vi "Set Struct Transfer Mode.vi"(8 "error in":errorcluster, 10 "Allow struct tranfer (False)":bool, 11 "GOLPI ref. in":T1={"pipe handle"={"lv_proc.dll file path"=path "", "process instance handle"=[], "debug mode"=FALSE, "debug data"=[]}, "fast read timeout [ms]"=500, "fast read settle time [ms]"=10, "fast read to multiple [ms]"=1, "max elements per input line"=100, "slow read timeout [ms]"=5000, "stdin double format specifier"="", "max elements per stdout output column"=100, "console mode bitstream"=FALSE, "bitstream first read timeout [ms]"=1000, "bitstream read timeout [ms]"=50, "struct transfer possible"=FALSE}) -> (0 "error out":errorcluster, 2 "conv struct possible?":bool, 3 "GOLPI ref. out":T1={"pipe handle"={"lv_proc.dll file path"=path "", "process instance handle"=[], "debug mode"=FALSE, "debug data"=[]}, "fast read timeout [ms]"=500, "fast read settle time [ms]"=10, "fast read to multiple [ms]"=1, "max elements per input line"=100, "slow read timeout [ms]"=5000, "stdin double format specifier"="", "max elements per stdout output column"=100, "console mode bitstream"=FALSE, "bitstream first read timeout [ms]"=1000, "bitstream read timeout [ms]"=50, "struct transfer possible"=FALSE})   [LabVIEW 2013, in "GOLPI library.lvlib"]
doc: "Set structure transfer mode. This is required for transfering of GNU Octave structures into LabVIEW cluster. First this VI tries to install GNU Octave package golpi. Than package is loaded and VI checks if function golpi_conv_struct() is available in current GNU Octave instance. If not the VIs related to structure tranfer will generate errors. This VI must be called before the structure transfer VIs can be used.\n\n---\nGOLPI works only with lv_proc.dll library, which is part of vipm package or should be delivered together with packed library. Placement of this dll is selected in terminal of Start GNU Octave.vi."
uses:
  GOLPI library.lvlib
  GOLPI reference Type Def.ctl
  LV Process source distribution/Pipe Handle.ctl
  Private/Type Definitions/Custom Error Codes Enum Type Def.vi
  <vilib>/regexp/Match Regular Expression.xnode
  LV Process source distribution/LV Process library.lvlib
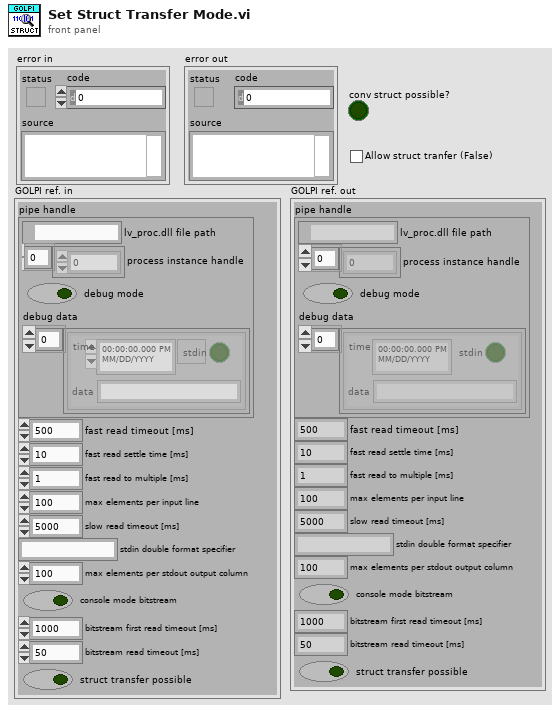
[diagram p1: front panel]
types:
  T1 = typedef "GOLPI library.lvlib/GOLPI reference Type Def.ctl" = cluster{"pipe handle":T2, "fast read timeout [ms]":u32, "fast read settle time [ms]":u32, "fast read to multiple [ms]":u32, "max elements per input line":u32, "slow read timeout [ms]":u32, "stdin double format specifier":string, "max elements per stdout output column":u32, "console mode bitstream":bool, "bitstream first read timeout [ms]":u32, "bitstream read timeout [ms]":u32, "struct transfer possible":bool}
  T2 = typedef "LV Process library.lvlib/Pipe Handle.ctl" = cluster{"lv_proc.dll file path":path, "process instance handle":u32[], "debug mode":bool, "debug data":cluster{"time":timestamp, "stdin":bool, "data":string}[]}
  T3 = typedef "GOLPI library.lvlib/Custom Error Codes Enum Type Def.vi" = enum16{"no error", "00 working directory PAR1 missing", "01 octave binary PAR1 missing", "02 octave report error PAR1", "03 empty output last cmd PAR1", "04 missing temporary file PAR1", "05 pwd PAR 1 not exist", "06 oct package not installed", "10 var PAR1 not string, vect", "11 var PAR1 not num, scal, ~compl", "12 var PAR1 not num, scal, compl", "13 var PAR1 not num, vect, ~compl", "14 var PAR1 not num, vect, compl", "15 var PAR1 not num, mat, ~compl", "16 var PAR1 not num, mat, ~compl", "30 read timeout", "60 bitstream transport failed", "61 bitstream decode error PAR1", "62 bitstream cannot be set", "70 struct transfer not possible", "80 struct: cluster elem. PAR1 not implem.", "81 struct: structure field PAR1 not implem.", "82 struct: size mismatch of PAR1", "83 struct: type mismatch of PAR1", "98 internal error", "99 not finished"}
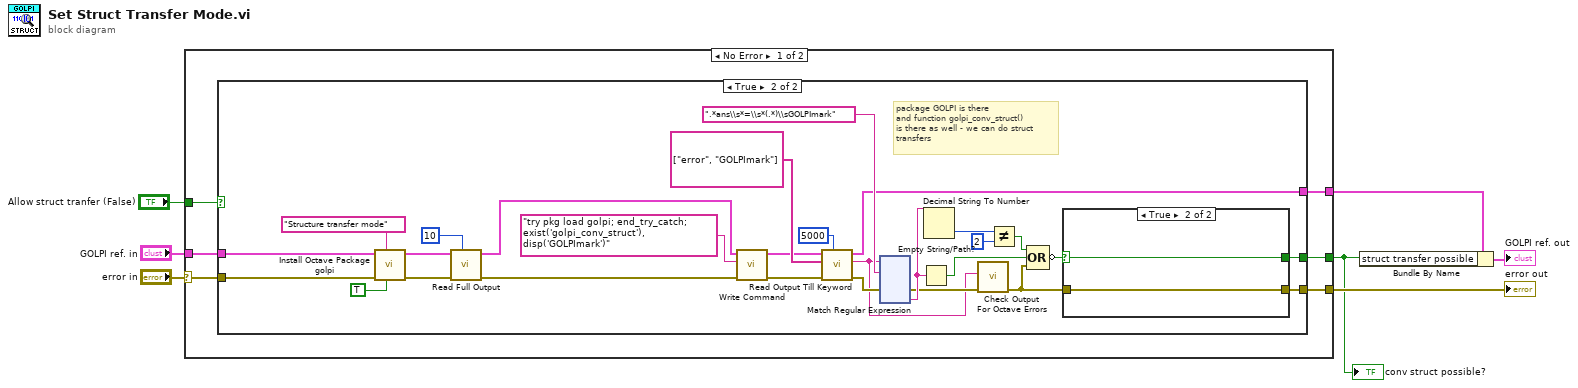
[diagram p0: block diagram]
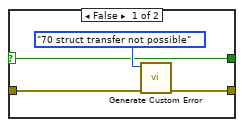
[diagram p3: hidden frame]
diagram:
  n1 = case shown="No Error" "error in" {
    selector: "error in" -> [w12 w167]
    tunnel: "GOLPI ref. in" -> [w13 w166]
    tunnel: [w11 w167] -> w5
    tunnel: [w10 w166] -> w3
    tunnel: [w9 _] -> w2
    tunnel: "Allow struct tranfer (False)" -> [w8 _]
    frame No Error {
      n2 = case shown="True" w8 {
        tunnel: w13 -> [w14 w19]
        tunnel: w12 -> [w15 w18]
        tunnel: [w15 w24] -> w11
        tunnel: [w14 w26] -> w10
        tunnel: [_ w22] -> w9
        frame False {
        }
        frame True {
          # "package GOLPI is there\nand function golpi_conv_struct()\nis there as well - we can do struct\ntransfers"
          n3 = call "Install Octave Package golpi.vi"("Verbose? (T)"=TRUE, "Feature name"="Structure transfer mode", "error in"=w18, "GOLPI ref. in"=w19) -> ("error out"=w17:errorcluster, "GOLPI ref. out"=w16:T1)  [unwired: 6 in]
          n4 = call "Read Full Output.vi"("timeout [ms]"=u32 10, "error in"=w17, "GOLPI ref. in"=w16) -> ("error out"=w42:errorcluster, "GOLPI ref. out"=w43:T1)  [unwired: 5 in, 2 out]
          n5 = call "Write Command.vi"("error in"=w42, "command"="try pkg load golpi; end_try_catch; exist('golpi_conv_struct'), disp('GOLPImark')", "GOLPI ref. in"=w43) -> ("error out"=w33:errorcluster, "GOLPI ref. out"=w31:T1)  [unwired: 7 in]
          n6 = call "Read Output Till Keyword.vi"("timeout [ms]"=u32 5000, "error in"=w33, "keywords"=string[] ["error", "GOLPImark"], "GOLPI ref. in"=w31) -> ("error out"=w32:errorcluster, "read buffer"=w27:string, "GOLPI ref. out"=w26:T1)  [unwired: 4 in, 1 out]
          n7 = xnode "Match Regular Expression"("input string"=w27, "regular expression"=".*ans\\s*=\\s*(.*)\\sGOLPImark", "error in"=w32) -> ("error out"=w34:errorcluster, "submatch 1"=w37:string)  [unwired: 3 in, 4 out]
          n8 = Empty String/Path?(string/path=w37) -> (empty?=w38:bool)
          n9 = Decimal String To Number(string=w37) -> (number=w28:i32)  [unwired: 2 in, 1 out]
          n10 = call "Check Output For Octave Errors.vi"("error in"=w34, "read buffer"=w27) -> ("error out"=w25:errorcluster)  [unwired: 9 in]
          n11 = Not Equal?(x=w28, y=2) -> (x != y?=w35:bool)
          n12 = Compound Arithmetic op=OR(w35, w38, w25) -> (invert w23:bool)
          n13 = case shown="True" w23 {
            selector: w23 -> [w44 w48]
            tunnel: w25 -> [w47 w49]
            tunnel: [w46 w49] -> w24
            tunnel: [w44 w48] -> w22
            frame False {
              n14 = call "Generate Custom Error.vi"("error in"=w47, "GOLPI error"=Custom_Error_Codes_Enum_Type_Def.vi."70 struct transfer not possible") -> ("error out"=w46:errorcluster)  [unwired: 9 in]
            }
            frame True {
            }
          }
        }
      }
    }
    frame Error {
    }
  }
  "error out" <- w5
  "conv struct possible?" <- w2
  n15 = Bundle By Name(cluster=w3, "struct transfer possible"=w2) -> (→"GOLPI ref. out":T1)
